vi "FormatMQTTPacket.vi"(7 "PacketFormatter":refnum<class "PacketFormatter.lvclass">, 10 "packet":T1) -> (2 "String":string)   [LabVIEW 2013, in "MQTT Base.lvlib" / "PacketFormatter.lvclass"]
uses:
  PacketFormatter.lvclass
  DebuggingTerminal/Packet Arrival -- cluster.ctl
  <vilib>/LabVIEW Open Source Project/MQTT Control Packets/Control Packets/ControlPacket/ControlPacket.lvclass
  DebuggingTerminal/DebuggingTerminal.lvclass
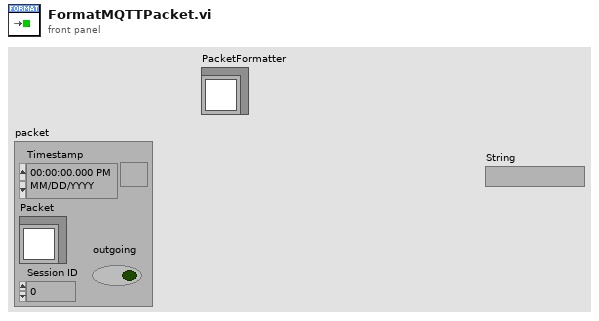
[diagram p1: front panel]
types:
  T1 = typedef "MQTT Base.lvlib/DebuggingTerminal.lvclass/Packet Arrival -- cluster.ctl" = cluster{"Timestamp":timestamp, "Packet":refnum<class "ControlPacket.lvclass">, "Session ID":i32, "outgoing":bool}
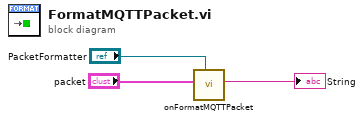
[diagram p0: block diagram]
diagram:
  n1 = call-dynamic "onFormatMQTTPacket.vi"("PacketFormatter"="PacketFormatter", "packet"="packet") -> ("String"=→"String":string)  [unwired: 9 in]
